vi "HFRR ADV v11.vi"() -> ()   [LabVIEW 2025] (continued)
                  n3634 = property on="TITTLE" class="Str"("Caption.Text"=w4919) -> ()  [unwired: 2 in, 2 out]
                }
                frame 109 {
                  "String 30" <- w4920
                }
                frame 110 {
                  n3635 = property on="Test Date" class="Str"("Caption.Text"=w4921) -> ()  [unwired: 2 in, 2 out]
                  "String 31" <- w4921
                }
                frame 111 {
                  n3636 = property on="Sample ID" class="Str"("Caption.Text"=w4922) -> ()  [unwired: 2 in, 2 out]
                  "String 32" <- w4922
                }
                frame 112 {
                  n3637 = property on="Tested by" class="Str"("Caption.Text"=w4923) -> ()  [unwired: 2 in, 2 out]
                  "String 33" <- w4923
                }
                frame 113 {
                  n3638 = property on="System Configured Printers 2" class="Arr (strict)"("Caption.Text"=w4924) -> ()  [unwired: 2 in, 2 out]
                }
                frame 114 {
                  n3639 = property on="Selected Printer" class="Str"("Caption.Text"=w4925) -> ()  [unwired: 2 in, 2 out]
                }
                frame 115 {
                  n3640 = property on="Select Printer 3" class="DigNum (strict)"("Caption.Text"=w4926) -> ()  [unwired: 2 in, 2 out]
                }
                frame 116 {
                  n3641 = property on="Print" class="Bool (strict)"("Boolean Text.Text"=w4927) -> ()  [unwired: 2 in, 2 out]
                }
                frame 117 {
                  "String 41" <- w4928
                }
                frame 118 {
                  n3642 = property on="tested by" class="Str"("Caption.Text"=w4929) -> ()  [unwired: 2 in, 2 out]
                }
                frame 119 {
                }
                frame 120 {
                  n3643 = property on="Export" class="Bool (strict)"("Boolean Text.Text"=w4930) -> ()  [unwired: 2 in, 2 out]
                }
                frame 121 {
                  n3644 = property on="TEMP INTERCEPT:" class="DigNum (strict)"("Caption.Text"=w4931) -> ()  [unwired: 2 in, 2 out]
                }
                frame 122 {
                  n3645 = property on="AIR TEMP INTERCEPT:" class="DigNum (strict)"("Caption.Text"=w4932) -> ()  [unwired: 2 in, 2 out]
                }
                frame 123 {
                  n3646 = property on="Select File Type" class="Enum (strict)"("Caption.Text"=w4933) -> ()  [unwired: 2 in, 2 out]
                }
                frame 124 {
                  n3647 = property on="s.NO" class="Str"("Caption.Text"=w4934) -> ()  [unwired: 2 in, 2 out]
                  "String 45" <- w4934
                }
                frame 125 {
                  n3648 = property on="trip1 8" class="Bool (strict)"("Boolean Text.Text"=w4935) -> ()  [unwired: 2 in, 2 out]
                }
                frame 126, Default {
                }
              }
            }
          }
          frame #1 {
            w4943 = TRUE ("Visible")
            n3649 = local read "S 91"() -> (w4960:string)
            n3650 = local read "S 90"() -> (w4959:string)
            n3651 = local read "S 88"() -> (w4958:string)
            n3652 = property on="Threshold" class="DigNum (strict)"("Caption.Text"=w4960) -> ()  [unwired: 2 in, 2 out]
            n3653 = property on="File Path" class="Path"("Caption.Text"=w4959) -> ()  [unwired: 2 in, 2 out]
            n3654 = property on="SrvM CP" class="Bool (strict)"("Boolean Text.Text"=w4958) -> ()  [unwired: 2 in, 2 out]
            n3655 = local read "S 71"() -> (w4953:string)
            n3656 = local read "S 86"() -> (w4955:string)
            n3657 = local read "S 85"() -> (w4956:string)
            n3658 = local read "S 87"() -> (w4954:string)
            n3659 = local read "S 84"() -> (w4957:string)
            n3660 = local read "S 103"() -> (w4942:string)
            n3661 = local read "S 104"() -> (w4941:string)
            n3662 = property on="ENTER THE NEW PASSWORD" class="Str"("Caption.Text"=w4954) -> ()  [unwired: 2 in, 2 out]
            n3663 = property on="Password" class="Str"("Caption.Text"=w4956) -> ()  [unwired: 2 in, 2 out]
            n3664 = property on="ENTER CURRENT PASSWORD" class="Str"("Caption.Text"=w4955) -> ()  [unwired: 2 in, 2 out]
            n3665 = property on="EDIT" class="Bool (strict)"("Boolean Text.Text"=w4953) -> ()  [unwired: 2 in, 2 out]
            n3666 = property on="SAVE" class="Bool (strict)"("Boolean Text.Text"=w4957) -> ()  [unwired: 2 in, 2 out]
            n3667 = Build Array(w4942, w4941) -> (w4940:string[])
            n3668 = property on="Heater Button" class="Bool (strict)"("Strings [4]"=w4940) -> ()  [unwired: 2 in, 2 out]
            n3669 = property on="CH-HUMIDITY WET" class="DigNum (strict)"("Caption.Size to Text?"=w4943) -> ()  [unwired: 2 in, 2 out]
            n3670 = property on="CH-HUMIDITY DRY" class="DigNum (strict)"("Caption.Size to Text?"=w4943) -> ()  [unwired: 2 in, 2 out]
            n3671 = property on="CH-POWER -" class="DigNum (strict)"("Caption.Size to Text?"=w4943) -> ()  [unwired: 2 in, 2 out]
            n3672 = property on="CH-HEATER" class="DigNum (strict)"("Caption.Size to Text?"=w4943) -> ()  [unwired: 2 in, 2 out]
            n3673 = property on="CH-POWER +" class="DigNum (strict)"("Caption.Size to Text?"=w4943) -> ()  [unwired: 2 in, 2 out]
            n3674 = local read "S 92"() -> (w4952:string)
            n3675 = local read "S 93"() -> (w4951:string)
            n3676 = local read "S 105"() -> (w4938:string)
            n3677 = local read "S 106"() -> (w4937:string)
            n3678 = Build Array(w4952, w4951) -> ()  [unwired: 1 out]
            n3679 = Build Array(w4938, w4937) -> (w4939:string[])
            n3680 = local read "S 95"() -> (w4949:string)
            n3681 = local read "S 94"() -> (w4950:string)
            n3682 = local read "bs"() -> (w4965:string)
            n3683 = local read "as"() -> (w4966:string)
            n3684 = property on="Humidity" class="Bool (strict)"("Strings [4]"=w4939) -> ()  [unwired: 2 in, 2 out]
            n3685 = Concatenate Strings(w4965, "\r", w4966) -> ()  [unwired: 1 out]
            n3686 = property on="STROKE GAIN :" class="DigNum (strict)"("Caption.Text"=w4949) -> ()  [unwired: 2 in, 2 out]
            n3687 = property on="DISPLACEMENT :" class="DigNum (strict)"("Caption.Text"=w4950) -> ()  [unwired: 2 in, 2 out]
            n3688 = property on="Rh After" class="DigNum (strict)"("Caption.Size to Text?"=TRUE ("Caption.Size to Text")) -> ()  [unwired: 2 in, 2 out]
            n3689 = local read "S 48"() -> (w4989:string)
            n3690 = local read "S 50"() -> (w4987:string)
            n3691 = local read "S 51"() -> (w4986:string)
            n3692 = local read "S 49"() -> (w4988:string)
            n3693 = local read "S 52"() -> (w4985:string)
            n3694 = local read "as"() -> (w4970:string)
            n3695 = local read "bs"() -> (w4971:string)
            n3696 = local read "S 56"() -> (w4984:string)
            n3697 = local read "S 57"() -> (w4983:string)
            n3698 = local read "S 58"() -> (w4982:string)
            n3699 = local read "S 59"() -> (w4981:string)
            n3700 = property on="OPEN" class="Bool (strict)"("Boolean Text.Text"=w4985) -> ()  [unwired: 2 in, 2 out]
            n3701 = property on="OPEN 1" class="Bool (strict)"("Boolean Text.Text"=w4989) -> ()  [unwired: 2 in, 2 out]
            n3702 = property on="OPEN 2" class="Bool (strict)"("Boolean Text.Text"=w4988) -> ()  [unwired: 2 in, 2 out]
            n3703 = property on="OPEN 3" class="Bool (strict)"("Boolean Text.Text"=w4987) -> ()  [unwired: 2 in, 2 out]
            n3704 = property on="OPEN 4" class="Bool (strict)"("Boolean Text.Text"=w4986) -> ()  [unwired: 2 in, 2 out]
            n3705 = Concatenate Strings(w4971, "\r", w4970) -> ()  [unwired: 1 out]
            n3706 = local read "S 102"() -> (w4944:string)
            n3707 = property on="КОФ1" class="DigNum (strict)"("Caption.Text"=w4984) -> ()  [unwired: 2 in, 2 out]
            n3708 = local read "S 98"() -> (w4948:string)
            n3709 = local read "S 99"() -> (w4947:string)
            n3710 = local read "S 100"() -> (w4946:string)
            n3711 = local read "S 101"() -> (w4945:string)
            n3712 = property on="КОФ2" class="DigNum (strict)"("Caption.Text"=w4983) -> ()  [unwired: 2 in, 2 out]
            n3713 = property on="КОФ3" class="DigNum (strict)"("Caption.Text"=w4982) -> ()  [unwired: 2 in, 2 out]
            n3714 = property on="КОФ4" class="DigNum (strict)"("Caption.Text"=w4981) -> ()  [unwired: 2 in, 2 out]
            n3715 = local read "bs"() -> (w4969:string)
            n3716 = local read "as"() -> (w4968:string)
            n3717 = property on="CH-POWER +" class="DigNum (strict)"("Caption.Text"=w4948) -> ()  [unwired: 2 in, 2 out]
            n3718 = property on="CH-POWER -" class="DigNum (strict)"("Caption.Text"=w4947) -> ()  [unwired: 2 in, 2 out]
            n3719 = property on="CH-HEATER" class="DigNum (strict)"("Caption.Text"=w4946) -> ()  [unwired: 2 in, 2 out]
            n3720 = property on="CH-HUMIDITY DRY" class="DigNum (strict)"("Caption.Text"=w4945) -> ()  [unwired: 2 in, 2 out]
            n3721 = property on="CH-HUMIDITY WET" class="DigNum (strict)"("Caption.Text"=w4944) -> ()  [unwired: 2 in, 2 out]
            n3722 = local read "S 60"() -> (w4980:string)
            n3723 = local read "S 54"() -> (w4990:string)
            n3724 = Concatenate Strings(w4969, "\r", w4968) -> ()  [unwired: 1 out]
            n3725 = Concatenate Strings(w4990, w4980) -> ()  [unwired: 1 out]
            n3726 = local read "S 77"() -> (→"String 43":string)
            n3727 = local read "S 76"() -> (w4963:string)
            n3728 = local read "S 78"() -> (w4962:string)
            n3729 = local read "S 71"() -> (w4974:string)
            n3730 = local read "S 66"() -> (w4979:string)
            n3731 = local read "S 67"() -> (w4978:string)
            n3732 = local read "S 68"() -> (w4977:string)
            n3733 = local read "S 69"() -> (w4976:string)
            n3734 = local read "S 70"() -> (w4975:string)
            n3735 = property on="AIR TEMP" class="DigNum (strict)"("Caption.Text"=w4962) -> ()  [unwired: 2 in, 2 out]
            n3736 = property on="Set Strk" class="DigNum (strict)"("Caption.Text"=w4963) -> ()  [unwired: 2 in, 2 out]
            n3737 = property on="FRIC. FORCE :" class="DigNum (strict)"("Caption.Text"=w4979) -> ()  [unwired: 2 in, 2 out]
            n3738 = property on="TEMPERATURE :" class="DigNum (strict)"("Caption.Text"=w4978) -> ()  [unwired: 2 in, 2 out]
            n3739 = property on="SPEED OUT:" class="DigNum (strict)"("Caption.Text"=w4977) -> ()  [unwired: 2 in, 2 out]
            n3740 = property on="AIR TEMPERATURE :" class="DigNum (strict)"("Caption.Text"=w4976) -> ()  [unwired: 2 in, 2 out]
            n3741 = property on="HUMIDITY:" class="DigNum (strict)"("Caption.Text"=w4975) -> ()  [unwired: 2 in, 2 out]
            n3742 = property on="EDIT" class="Bool (strict)"("Boolean Text.Text"=w4974) -> ()  [unwired: 2 in, 2 out]
            n3743 = local read "S 79"() -> (w4961:string)
            n3744 = property on="Stroke" class="DigNum (strict)"("Caption.Text"=w4961) -> ()  [unwired: 2 in, 2 out]
          }
          frame #2 {
          }
        }
        n3745 = local write "Lan flag"(10.0 ("Lan flag")) -> ()
      }
      frame Enabled {
      }
    }
    n3746 = Wait (ms)(milliseconds to wait=u32 2000) -> ()  [unwired: 1 out]
    n3747 = local read "Quit"() -> (w4763:bool)
  }
  n3748 = disable-structure shown="Disabled" {
    frame Disabled {
      n3749 = while {
        tunnel: [w4992] -> _
        i -> [w4992]
        stop <- w4991 continue-if-true
        n3750 = Wait (ms)(milliseconds to wait=u32 50) -> ()  [unwired: 1 out]
        n3751 = stacked-sequence {
          frame #0 {
            # "Controls Text color"
            # "Controls BG color"
            n3752 = property on="FILE" class="Str"("Text.Text Colors:Text Color"="SC  Text") -> ()  [unwired: 2 in, 2 out]
            n3753 = property on="Fuel Discription :" class="Str"("Text.Text Colors:Text Color"="SC  Text") -> ()  [unwired: 2 in, 2 out]
            n3754 = property on="tested by" class="Str"("Text.Text Colors:Text Color"="SC  Text") -> ()  [unwired: 2 in, 2 out]
            n3755 = property on="Remarks :" class="Str"("Text.Text Colors:Text Color"="SC  Text") -> ()  [unwired: 2 in, 2 out]
            n3756 = property class="DigNum (strict)"("Numeric Text.Text Colors:BG Color"="NC BG") -> ()  [unwired: 2 in, 2 out]
            n3757 = property class="DigNum (strict)"("Numeric Text.Text Colors:BG Color"="NC BG") -> ()  [unwired: 2 in, 2 out]
            n3758 = property class="DigNum (strict)"("Numeric Text.Text Colors:BG Color"="NC BG") -> ()  [unwired: 2 in, 2 out]
            n3759 = property class="DigNum (strict)"("Numeric Text.Text Colors:BG Color"="NC BG") -> ()  [unwired: 2 in, 2 out]
            n3760 = property class="DigNum (strict)"("Numeric Text.Text Colors:BG Color"="NC BG") -> ()  [unwired: 2 in, 2 out]
            n3761 = property class="DigNum (strict)"("Numeric Text.Text Colors:BG Color"="NC BG") -> ()  [unwired: 2 in, 2 out]
            n3762 = property class="DigNum (strict)"("Numeric Text.Text Colors:BG Color"="NC BG") -> ()  [unwired: 2 in, 2 out]
            n3763 = property class="DigNum (strict)"("Numeric Text.Text Colors:BG Color"="NC BG") -> ()  [unwired: 2 in, 2 out]
            n3764 = property class="DigNum (strict)"("Numeric Text.Text Colors:BG Color"="NC BG") -> ()  [unwired: 2 in, 2 out]
            n3765 = property class="DigNum (strict)"("Numeric Text.Text Colors:BG Color"="NC BG") -> ()  [unwired: 2 in, 2 out]
            n3766 = property class="DigNum (strict)"("Numeric Text.Text Colors:BG Color"="NC BG") -> ()  [unwired: 2 in, 2 out]
            n3767 = property class="DigNum (strict)"("Numeric Text.Text Colors:BG Color"="NC BG") -> ()  [unwired: 2 in, 2 out]
            n3768 = property on="FILE" class="Str"("Text.Text Colors:BG Color"="SC BG 3") -> ()  [unwired: 2 in, 2 out]
            n3769 = property on="Fuel Discription :" class="Str"("Text.Text Colors:BG Color"="SC BG 3") -> ()  [unwired: 2 in, 2 out]
            n3770 = property on="tested by" class="Str"("Text.Text Colors:BG Color"="SC BG 3") -> ()  [unwired: 2 in, 2 out]
            n3771 = property on="Remarks :" class="Str"("Text.Text Colors:BG Color"="SC BG 3") -> ()  [unwired: 2 in, 2 out]
            n3772 = property class="DigNum (strict)"("Numeric Text.Text Colors:Text Color"="NC Text") -> ()  [unwired: 2 in, 2 out]
            n3773 = property class="DigNum (strict)"("Numeric Text.Text Colors:Text Color"="NC Text") -> ()  [unwired: 2 in, 2 out]
            n3774 = property class="DigNum (strict)"("Numeric Text.Text Colors:Text Color"="NC Text") -> ()  [unwired: 2 in, 2 out]
            n3775 = property class="DigNum (strict)"("Numeric Text.Text Colors:Text Color"="NC Text") -> ()  [unwired: 2 in, 2 out]
            n3776 = property class="DigNum (strict)"("Numeric Text.Text Colors:Text Color"="NC Text") -> ()  [unwired: 2 in, 2 out]
            n3777 = property class="DigNum (strict)"("Numeric Text.Text Colors:Text Color"="NC Text") -> ()  [unwired: 2 in, 2 out]
            n3778 = property class="DigNum (strict)"("Numeric Text.Text Colors:Text Color"="NC Text") -> ()  [unwired: 2 in, 2 out]
            n3779 = property class="DigNum (strict)"("Numeric Text.Text Colors:Text Color"="NC Text") -> ()  [unwired: 2 in, 2 out]
            n3780 = property class="DigNum (strict)"("Numeric Text.Text Colors:Text Color"="NC Text") -> ()  [unwired: 2 in, 2 out]
            n3781 = property class="DigNum (strict)"("Numeric Text.Text Colors:Text Color"="NC Text") -> ()  [unwired: 2 in, 2 out]
            n3782 = property class="DigNum (strict)"("Numeric Text.Text Colors:Text Color"="NC Text") -> ()  [unwired: 2 in, 2 out]
            n3783 = property class="DigNum (strict)"("Numeric Text.Text Colors:Text Color"="NC Text") -> ()  [unwired: 2 in, 2 out]
            n3784 = property class="DigNum (strict)"("Numeric Text.Text Colors:Text Color"="NI Text  2") -> ()  [unwired: 2 in, 2 out]
            n3785 = property class="DigNum (strict)"("Numeric Text.Text Colors:Text Color"="NI Text  2") -> ()  [unwired: 2 in, 2 out]
            n3786 = property class="DigNum (strict)"("Numeric Text.Text Colors:Text Color"="NI Text  2") -> ()  [unwired: 2 in, 2 out]
            n3787 = property class="DigNum (strict)"("Numeric Text.Text Colors:Text Color"="NI Text  2") -> ()  [unwired: 2 in, 2 out]
            n3788 = property class="DigNum (strict)"("Numeric Text.Text Colors:Text Color"="NI Text  2") -> ()  [unwired: 2 in, 2 out]
            n3789 = property class="DigNum (strict)"("Numeric Text.Text Colors:Text Color"="NI Text  2") -> ()  [unwired: 2 in, 2 out]
            n3790 = property class="DigNum (strict)"("Numeric Text.Text Colors:Text Color"="NI Text  2") -> ()  [unwired: 2 in, 2 out]
            n3791 = property class="DigNum (strict)"("Numeric Text.Text Colors:Text Color"="NI Text  2") -> ()  [unwired: 2 in, 2 out]
            n3792 = property class="DigNum (strict)"("Numeric Text.Text Colors:Text Color"="NI Text  2") -> ()  [unwired: 2 in, 2 out]
            n3793 = property class="DigNum (strict)"("Numeric Text.Text Colors:Text Color"="NI Text  2") -> ()  [unwired: 2 in, 2 out]
            n3794 = property class="DigNum (strict)"("Numeric Text.Text Colors:Text Color"="NI Text  2") -> ()  [unwired: 2 in, 2 out]
            n3795 = property class="DigNum (strict)"("Numeric Text.Text Colors:Text Color"="NI Text  2") -> ()  [unwired: 2 in, 2 out]
            n3796 = property class="DigNum (strict)"("Numeric Text.Text Colors:Text Color"="NI Text  2") -> ()  [unwired: 2 in, 2 out]
            n3797 = property class="DigNum (strict)"("Numeric Text.Text Colors:Text Color"="NI Text  2") -> ()  [unwired: 2 in, 2 out]
            n3798 = property class="DigNum (strict)"("Numeric Text.Text Colors:Text Color"="NI Text  2") -> ()  [unwired: 2 in, 2 out]
            n3799 = property class="DigNum (strict)"("Numeric Text.Text Colors:Text Color"="NI Text  2") -> ()  [unwired: 2 in, 2 out]
            n3800 = property on="Coefficient Of Friction" class="XYGraph (strict)"("Plot Area:Colors:FG Color"="GFG  2", "Plot Area:Colors:BG Color"="GBG   2") -> ()  [unwired: 2 in, 2 out]
            n3801 = property on="Humidity ( %RH )" class="XYGraph (strict)"("Plot Area:Colors:FG Color"="GFG  2", "Plot Area:Colors:BG Color"="GBG   2") -> ()  [unwired: 2 in, 2 out]
            n3802 = property on="Air Temperature  ( °C )" class="XYGraph (strict)"("Plot Area:Colors:FG Color"="GFG  2", "Plot Area:Colors:BG Color"="GBG   2") -> ()  [unwired: 2 in, 2 out]
            n3803 = property on="Sample Temperature ( °C )" class="XYGraph (strict)"("Plot Area:Colors:FG Color"="GFG  2", "Plot Area:Colors:BG Color"="GBG   2") -> ()  [unwired: 2 in, 2 out]
            n3804 = property class="DigNum (strict)"("Numeric Text.Text Colors:BG Color"="NI BG 2") -> ()  [unwired: 2 in, 2 out]
            n3805 = property class="DigNum (strict)"("Numeric Text.Text Colors:BG Color"="NI BG 2") -> ()  [unwired: 2 in, 2 out]
            n3806 = property class="DigNum (strict)"("Numeric Text.Text Colors:BG Color"="NI BG 2") -> ()  [unwired: 2 in, 2 out]
            n3807 = property class="DigNum (strict)"("Numeric Text.Text Colors:BG Color"="NI BG 2") -> ()  [unwired: 2 in, 2 out]
            n3808 = property class="DigNum (strict)"("Numeric Text.Text Colors:BG Color"="NI BG 2") -> ()  [unwired: 2 in, 2 out]
            n3809 = property class="DigNum (strict)"("Numeric Text.Text Colors:BG Color"="NI BG 2") -> ()  [unwired: 2 in, 2 out]
            n3810 = property class="DigNum (strict)"("Numeric Text.Text Colors:BG Color"="NI BG 2") -> ()  [unwired: 2 in, 2 out]
            n3811 = property class="DigNum (strict)"("Numeric Text.Text Colors:BG Color"="NI BG 2") -> ()  [unwired: 2 in, 2 out]
            n3812 = property class="DigNum (strict)"("Numeric Text.Text Colors:BG Color"="NI BG 2") -> ()  [unwired: 2 in, 2 out]
            n3813 = property class="DigNum (strict)"("Numeric Text.Text Colors:BG Color"="NI BG 2") -> ()  [unwired: 2 in, 2 out]
            n3814 = property class="DigNum (strict)"("Numeric Text.Text Colors:BG Color"="NI BG 2") -> ()  [unwired: 2 in, 2 out]
            n3815 = property class="DigNum (strict)"("Numeric Text.Text Colors:BG Color"="NI BG 2") -> ()  [unwired: 2 in, 2 out]
            n3816 = property class="DigNum (strict)"("Numeric Text.Text Colors:BG Color"="NI BG 2") -> ()  [unwired: 2 in, 2 out]
            n3817 = property class="DigNum (strict)"("Numeric Text.Text Colors:BG Color"="NI BG 2") -> ()  [unwired: 2 in, 2 out]
            n3818 = property class="DigNum (strict)"("Numeric Text.Text Colors:BG Color"="NI BG 2") -> ()  [unwired: 2 in, 2 out]
            n3819 = property class="DigNum (strict)"("Numeric Text.Text Colors:BG Color"="NI BG 2") -> ()  [unwired: 2 in, 2 out]
            n3820 = property class="Bool"("Colors [4]"="Boolean BC T & BG") -> ()  [unwired: 2 in, 2 out]
            n3821 = property on="Save & Continue" class="Bool (strict)"("Colors [4]"="Boolean BC T & BG") -> ()  [unwired: 2 in, 2 out]
            n3822 = property on="Heater Button" class="Bool (strict)"("Colors [4]"="Boolean BC T & BG") -> ()  [unwired: 2 in, 2 out]
            n3823 = property class="Bool"("Colors [4]"="Boolean BC T & BG") -> ()  [unwired: 2 in, 2 out]
            n3824 = property on="Humidity" class="Bool (strict)"("Colors [4]"="Boolean BC T & BG") -> ()  [unwired: 2 in, 2 out]
            n3825 = property class="Bool (strict)"("Colors [4]"="Boolean BC T & BG") -> ()  [unwired: 2 in, 2 out]
            n3826 = property on="RUN" class="Bool (strict)"("Colors [4]"="Boolean BC T & BG") -> ()  [unwired: 2 in, 2 out]
            n3827 = property on="trip1 8" class="Bool (strict)"("Colors [4]"="Boolean BC T & BG") -> ()  [unwired: 2 in, 2 out]
            n3828 = property class="Bool"("Colors [4]"="Boolean BC T & BG") -> ()  [unwired: 2 in, 2 out]
            n3829 = property class="Bool (strict)"("Colors [4]"="Boolean BC T & BG") -> ()  [unwired: 2 in, 2 out]
            n3830 = property on="OPEN 1" class="Bool (strict)"("Colors [4]"="Boolean BC T & BG 2") -> ()  [unwired: 2 in, 2 out]
            n3831 = property on="OPEN 2" class="Bool (strict)"("Colors [4]"="Boolean BC T & BG 2") -> ()  [unwired: 2 in, 2 out]
            n3832 = property on="OPEN 3" class="Bool (strict)"("Colors [4]"="Boolean BC T & BG 2") -> ()  [unwired: 2 in, 2 out]
            n3833 = property on="OPEN 4" class="Bool (strict)"("Colors [4]"="Boolean BC T & BG 2") -> ()  [unwired: 2 in, 2 out]
            n3834 = property on="OPEN" class="Bool (strict)"("Colors [4]"="Boolean BC T & BG 2") -> ()  [unwired: 2 in, 2 out]
            n3835 = property on="rstv2" class="Bool"("Colors [4]"="Boolean BC T & BG 2") -> ()  [unwired: 2 in, 2 out]
            n3836 = property on="RST CP" class="Bool"("Colors [4]"="Boolean BC T & BG 2") -> ()  [unwired: 2 in, 2 out]
            n3837 = property on="RSTV1 3" class="Bool"("Colors [4]"="Boolean BC T & BG 2") -> ()  [unwired: 2 in, 2 out]
            n3838 = property on="RSTV1 2" class="Bool"("Colors [4]"="Boolean BC T & BG 2") -> ()  [unwired: 2 in, 2 out]
          }
          frame #1 {
          }
        }
        n3839 = local read "Quit"() -> (w4991:bool)
      }
    }
    frame Enabled {
    }
  }
  n3840 = while {
    shift-right: [w5009] -> _
    shift-left: _ -> [w5010]
    shift-right: [w5007] -> _
    shift-left: T17 {"Read Heave and Surge"="", "Bytes at Heave Port"=0.0, "Heave and Surge COM Port:"="COM9", "Com Port 2"="COM7", "Residual Due"="", "Heave COM Status 2"=TRUE, "Heave COM Status"=TRUE, "Port 2"=TRUE, "Sway PPR"=6400.0, "Surge PPR"=6400.0, "Heave PPR"=6400.0, "Sway Pitch"=2.0, "Surge Pitch"=3.0, "Heave Pitch"=4.0, "Sway Pulses/mm"=320.0, "Surge Pulses/mm"=1600.0, "Heave Pulses/mm"=1600.0, "inner loop"=0.0, "Read Heave and Surge 2"="", "String 36"="", "Write S"=FALSE, "WriteCC1"=[""], "Heave COM Loop"=0, "LastCom"="", "EXIT"=FALSE, "Error Heave"={"status"=TRUE, "code"=-1073807343, "source"=""}} -> [w5006]
    shift-right: [w5004] -> _
    shift-left: enum16{"init", "MAIN", "Panel Close"}."init" -> [w5005]
    stop <- w5008 stop-if-true
    n3841 = case shown="\"init\"" w5005 {
      tunnel: w5010 -> [w5024 w5039 w5109 w5111]
      tunnel: [w5018 w5057 w5109 w5111] -> w5009
      tunnel: [_ _ TRUE _] -> w5008
      tunnel: [w5014 w5054 w5107 w5110] -> w5007
      tunnel: w5006 -> [w5021 w5038 w5107 w5110]
      tunnel: [enum16{"init", "MAIN", "Panel Close"}."MAIN" w5032 _ _] -> w5004
      frame "init" {
        n3842 = Bundle By Name(cluster=w5021, "Heave and Surge COM Port:"="C3 :") -> (w5020:T17)
        n3843 = call "Instrument fgv.vi"("Enum"=T27."INIT", "error in (no error) 2"=w5024, "INPUT"=w5020) -> ("error"=w5022:errorcluster, "output"=w5017:T17)  [unwired: 6 in, 1 out]
        n3844 = case shown="No Error" w5022 {
          selector: w5022 -> [w5026 _]
          tunnel: [w5026 w5030] -> w5018
          tunnel: w5017 -> [w5025 w5028]
          tunnel: [w5025 w5027] -> w5015
          frame No Error {
          }
          frame Error {
            n3845 = call "Instrument fgv.vi"("Enum"=T27."ERROR INIT", "INPUT"=w5028) -> ("error"=w5031:errorcluster, "output"=w5027:T17)  [unwired: 7 in, 1 out]
            n3846 = call <vilib>:"Clear Errors.vi"("error in (no error)"=w5031) -> ("error out"=w5030:errorcluster)  [unwired: 5 in, 1 out]
          }
        }
        n3847 = local read "LastCom"() -> (w5013:string)
        n3848 = Unbundle By Name(w5015) -> ("Heave COM Status 2"=→"COM Status" →"Instrument Status":bool, "Error Heave"=→"Error":errorcluster)  [unwired: 1 out]
        n3849 = Bundle By Name(cluster=w5015, "LastCom"=w5013) -> (w5014:T17)
      }
      frame "MAIN" {
        n3850 = Unbundle By Name(w5038) -> ("Com Port 2"=w5059:refnum<visa-resource-name>)
        n3851 = local write "Com Port 4"(w5059) -> ()
        n3852 = local read "C3 :"() -> (w5036:refnum<visa-resource-name>)
        n3853 = Divide(x="Heave PPR", y="Heave Pitch") -> (x/y=→"Heave Pulses/mm":dbl)
        n3854 = Bundle By Name(cluster=w5038, "Heave and Surge COM Port:"=w5036) -> (w5037:T17)
        n3855 = Equal?(x=w5059, y=w5036) -> (x = y?=w5058:bool)
        n3856 = Divide(x="Sway PPR", y="Sway Pitch") -> (x/y=→"Sway Pulses/mm":dbl)
        n3857 = case shown="False" w5058 {
          tunnel: [w5063 w5080] -> w5057
          tunnel: w5039 -> [w5064 w5086]
          tunnel: w5037 -> [w5062 w5084]
          tunnel: [w5061 w5079] -> w5054
          frame False {
            n3858 = call <vilib>:"Clear Errors.vi"("error in (no error)"=w5064) -> ("error out"=w5060:errorcluster)  [unwired: 5 in, 1 out]
            n3859 = call "Instrument fgv.vi"("Enum"=T27."ERROR INIT", "error in (no error) 2"=w5060, "INPUT"=w5062) -> ("error"=w5066:errorcluster, "output"=w5061:T17)  [unwired: 6 in, 1 out]
            n3860 = call <vilib>:"Clear Errors.vi"("error in (no error)"=w5066) -> ("error out"=w5063:errorcluster)  [unwired: 5 in, 1 out]
          }
          frame True {
            n3861 = call "Instrument fgv.vi"("Enum"=T27."READ", "error in (no error) 2"=w5086, "INPUT"=w5084) -> ("error"=w5085:errorcluster, "output"=w5076:T17)  [unwired: 6 in, 1 out]
            n3862 = Bundle By Name(cluster=w5076, "String 36"="String 11") -> (w5075:T17)
            n3863 = case shown="True" "Write S" {
              selector: "Write S" -> [_ w5106]
              tunnel: w5085 -> [w5099 w5105]
              tunnel: [w5099 w5104] -> w5072
              tunnel: w5075 -> [w5098 w5101]
              tunnel: [w5098 w5100] -> w5071
              frame False {
              }
              frame True {
                n3864 = Not(x=w5106) -> (.not. x?=w5102:bool)
                n3865 = local write "Write S"(w5102) -> ()
                n3866 = call "Instrument fgv.vi"("Enum"=T27."MANUAL WRITE", "error in (no error) 2"=w5105, "INPUT"=w5101) -> ("error"=w5104:errorcluster, "output"=w5100:T17)  [unwired: 6 in, 1 out]
              }
            }
            n3867 = Array Size(array="WriteHumidity") -> (size(s)=w5069:i32)
            n3868 = Greater Than 0?(x=w5069) -> (x > 0?=w5067:bool)
            n3869 = call "Instrument fgv.vi"("Enum"=T27."WRITE", "error in (no error) 2"=w5072, "WriteCC1"="WriteHumidity", "INPUT"=w5071) -> ("error"=w5082:errorcluster, "WriteCC1 2"=w5070:string[], "output"=w5081:T17)  [unwired: 5 in]
            n3870 = case shown="True" w5067 {
              tunnel: w5070 -> [_ w5088]
              frame False {
              }
              frame True {
                n3871 = local write "WriteHumidity"(w5088) -> ()
              }
            }
            n3872 = case shown="Error" w5082 {
              selector: w5082 -> [w5089 w5092]
              tunnel: w5081 -> [w5090 w5097]
              tunnel: [w5090 w5096] -> w5079
              tunnel: [w5089 w5094] -> w5080
              frame No Error {
              }
              frame Error {
                n3873 = call <vilib>:"Clear Errors.vi"("error in (no error)"=w5092) -> ("error out"=w5091:errorcluster)  [unwired: 5 in, 1 out]
                n3874 = call "Instrument fgv.vi"("Enum"=T27."ERROR INIT", "error in (no error) 2"=w5091, "INPUT"=w5097) -> ("error"=w5095:errorcluster, "output"=w5096:T17)  [unwired: 6 in, 1 out]
                n3875 = call <vilib>:"Clear Errors.vi"("error in (no error)"=w5095) -> ("error out"=w5094:errorcluster)  [unwired: 5 in, 1 out]
              }
            }
            n3876 = Unbundle By Name(w5079) -> ("LastCom"=→"LastCom":string, "Read Heave and Surge"=→"Read Humidity":string)
          }
        }
        n3877 = Divide(x="Surge PPR", y="Surge Pitch") -> (x/y=→"Surge Pulses/mm":dbl)
        n3878 = Unbundle By Name(w5054) -> ("Heave COM Status 2"=w5056:bool, "Heave COM Status"=w5055:bool, "Error Heave"=w5052:errorcluster, "Bytes at Heave Port"=→"Bytes at Humidity Port":dbl)
        n3879 = Unbundle By Name(w5052) -> ("status"=→"Humidity Port":bool)
        n3880 = Not(x=w5055) -> (.not. x?=w5040:bool)
        n3881 = local write "Error"(w5052) -> ()
        n3882 = Not(x=w5056) -> (.not. x?=w5041:bool)
        n3883 = local write "Instrument Status"(w5040) -> ()
        n3884 = local write "COM Status"(w5041) -> ()
        n3885 = local read "Quit"() -> (w5033:bool)
        n3886 = Select(t=enum16{"init", "MAIN", "Panel Close"}."Panel Close", s=w5033, f=enum16{"init", "MAIN", "Panel Close"}."MAIN") -> (s? t:f=w5032:enum16{"init", "MAIN", "Panel Close"})
      }
      frame "Panel Close" {
      }
      frame Default {
      }
    }
  }
  n3887 = while {
    stop <- w5137 stop-if-true
    n3888 = local read "Read Humidity"() -> (w5118:string)
    n3889 = call <vilib>:"High Resolution Polling Wait.vi"("seconds to wait"=0.1) -> ()  [unwired: 10 in, 1 out]
    n3890 = Spreadsheet String To Array(delimiter (Tab)=",", format string="", spreadsheet string=w5118, array type (2D Dbl)=string[] []) -> (array=w5132:string[])
    n3891 = for {
      tunnel: w5132 -> [w5142] mode=indexing
      tunnel: string[] ["STATE;", "SET;", "RH;", "T;", "AMB_RH;", "AMB_T;", "PUMP;", "FAN_IN;", "FAN_OUT;", "DEHUM;", "CURRENT;", "STALL;"] -> [w5141] mode=indexing
      tunnel: [w5140] -> w5131 mode=indexing
      n3892 = Match Pattern(string=w5142, regular expression=w5141) -> (after substring=w5140:string)  [unwired: 1 in, 3 out]
    }
    n3893 = Index Array(array=w5131) -> (element #1=→"STATE :":string, element #2=→"SET :":string, element #3=w5120:string, element #4=→"T :":string, element #5=w5117:string, element #6=→"AMB_T :":string, element #7=→"PUMP :":string, element #8=→"FAN_IN :":string, element #9=→"FAN_OUT :":string, element #10=→"DEHUM :":string, element #11=→"CURRENT :":string, element #12=→"STALL :":string)  [unwired: 12 in]
    "RH :" <- w5120
    "AMB_RH :" <- w5117
    n3894 = Fract/Exp String To Number(string=w5120) -> (number=w5112:dbl)  [unwired: 3 in, 1 out]
    n3895 = Fract/Exp String To Number(string=w5117) -> (number=w5116:dbl)  [unwired: 3 in, 1 out]
    n3896 = local write "Ambient Humidity :"(w5116) -> ()
    n3897 = Equal?(x=w5112, y=0.0) -> (x = y?=w5114:bool)
    n3898 = case shown="True" w5114 {
      tunnel: [w5138 w5139] -> w5113
      tunnel: w5112 -> [w5138 _]
      frame False {
        (unwired) 0.0
        "Humidity temp" <- w5138
      }
      frame True {
        n3899 = local read "Humidity temp"() -> (w5139:dbl)
      }
    }
    "RH Numeric:" <- w5113
    n3900 = local read "Quit"() -> (w5137:bool)
  }
  n3901 = disable-structure shown="Disabled" {
    frame Disabled {
      n3902 = while {
        tunnel: [w5376] -> _
        i -> [w5376]
        stop <- w5373 stop-if-true
        n3903 = local read "powstat"() -> (w5374:bool)
        n3904 = case shown="True" w5374 {
          frame False {
          }
          frame True {
            n3905 = local read "RUN"() -> (w5377:bool)
            n3906 = case shown="True" w5377 {
              frame False {
                w5407 = 65.0 ("y")
                n3907 = local read "Set Hz"() -> (w5435:dbl)
                n3908 = local read "NORMAL LOAD"() -> (w5436:dbl)
                n3909 = Multiply(x=w5435, y=60.0) -> (x*y=w5442:dbl)
                n3910 = Multiply(x=1.2 ("y"), y=0.949) -> (x*y=w5411:dbl)
                n3911 = Multiply(x=1.2 ("y"), y=0.8166) -> (x*y=w5415:dbl)
                n3912 = Multiply(x=1.2 ("y"), y=0.851) -> (x*y=w5410:dbl)
                n3913 = local read "FF 2"() -> (w5434:dbl)
                n3914 = Absolute Value(x=w5442) -> (abs(x)=w5440:dbl)
                n3915 = local read "Stroke"() -> (w5409:dbl)
                n3916 = Less?(x=w5409, y=w5415) -> (x < y?=w5412:bool)
                n3917 = In Range and Coerce(upper limit=w5411, x=w5409, lower limit=w5410) -> (In Range?=w5413:bool)  [unwired: 1 out]
                n3918 = case shown="13.." w5434 {
                  tunnel: [1 2 3] -> w5432
                  frame 0..10, Default {
                    # "Normal"
                  }
                  frame 11, 12 {
                  }
                  frame 13.. {
                  }
                }
                "FF STATE" <- w5432
                n3919 = local read "TEMP"() -> (w5395:dbl)
                n3920 = case shown="3601.." w5440 {
                  tunnel: [1 2 3] -> w5438
                  frame 0..3000, Default {
                    # "Normal"
                  }
                  frame 3001..3600 {
                  }
                  frame 3601.. {
                  }
                }
                n3921 = case shown="11.." w5436 {
                  tunnel: [1 3] -> w5437
                  frame 1..10, Default {
                  }
                  frame 11.. {
                  }
                }
                "NL STATE" <- w5437
                n3922 = Multiply(x=1.2 ("y"), y=0.95) -> (x*y=w5425:dbl)
                n3923 = Multiply(x=w5407, y=0.954) -> (x*y=w5399:dbl)
                n3924 = Or(x=w5412, y=w5413) -> (x .or. y?=w5414:bool)
                n3925 = Greater Or Equal?(x=w5409, y=w5425) -> (x >= y?=w5422:bool)
                n3926 = Multiply(x=w5407, y=0.99) -> (x*y=w5396:dbl)
                n3927 = Greater Or Equal?(x=w5395, y=w5396) -> (x >= y?=w5401:bool)
                n3928 = Greater Or Equal?(x=w5395, y=w5399) -> (x >= y?=w5398:bool)
                n3929 = case shown="0, 1, Default" w5409 {
                  tunnel: [1 3] -> w5426
                  frame 0, 1, Default {
                  }
                  frame 2.. {
                  }
                }
                n3930 = case shown="True" w5422 {
                  tunnel: [1 3] -> w5427
                  frame False {
                  }
                  frame True {
                  }
                }
                n3931 = case shown="True" w5414 {
                  tunnel: [1 2] -> w5428
                  frame False {
                  }
                  frame True {
                  }
                }
                n3932 = case shown="..0" w5395 {
                  tunnel: [2 3 3 1] -> w5402
                  frame 61, 62 {
                  }
                  frame 63.. {
                  }
                  frame ..0 {
                  }
                  frame 10..60, Default {
                  }
                }
                n3933 = case shown="True" w5401 {
                  tunnel: [1 3] -> w5403
                  frame False {
                  }
                  frame True {
                  }
                }
                n3934 = Number To Decimal String(number=w5438) -> (decimal integer string=w5439:string)  [unwired: 1 in]
                n3935 = case shown="True" w5398 {
                  tunnel: [1 2] -> w5404
                  frame False {
                  }
                  frame True {
                  }
                }
                n3936 = Number To Decimal String(number=1) -> (decimal integer string=→"Air temp":string)  [unwired: 1 in]
                n3937 = Number To Decimal String(number=w5432) -> (decimal integer string=→"ff_st":string)  [unwired: 1 in]
                n3938 = local write "sp_st"(w5439) -> ()
                n3939 = Number To Decimal String(number=w5437) -> (decimal integer string=→"nl_st":string)  [unwired: 1 in]
                n3940 = Build Array(w5402, w5403, w5404) -> (w5405:i32[])
                n3941 = Build Array(w5426, w5427, w5428) -> (w5429:i32[])
                n3942 = Array Max & Min(array=w5405) -> (max value=w5406:i32)  [unwired: 3 out]
                n3943 = Array Max & Min(array=w5429) -> (max value=w5430:i32)  [unwired: 3 out]
                n3944 = Number To Decimal String(number=w5406) -> (decimal integer string=w5394:string)  [unwired: 1 in]
                n3945 = Number To Decimal String(number=w5430) -> (decimal integer string=→"Stroke Ln 2":string)  [unwired: 1 in]
                n3946 = local write "temp_st"(w5394) -> ()
              }
              frame True {
                w5492 = 65.0 ("y")
                # "Healthy -1\nWarning -2\nError -3"
                n3947 = local read "TEMP"() -> (w5503:dbl)
                n3948 = local read "NORMAL LOAD"() -> (w5507:dbl)
                n3949 = local read "Set Hz"() -> (w5505:dbl)
                n3950 = Multiply(x=1.2 ("y"), y=0.949) -> (x*y=w5487:dbl)
                n3951 = Multiply(x=1.2 ("y"), y=0.8166) -> (x*y=w5483:dbl)
                n3952 = Multiply(x=1.2 ("y"), y=0.851) -> (x*y=w5488:dbl)
                n3953 = Multiply(x=w5492, y=0.954) -> (x*y=w5499:dbl)
                n3954 = Multiply(x=w5492, y=0.99) -> (x*y=w5502:dbl)
                n3955 = Greater Or Equal?(x=w5503, y=w5502) -> (x >= y?=w5497:bool)
                n3956 = Multiply(x=w5505, y=60.0) -> (x*y=w5511:dbl)
                n3957 = Greater Or Equal?(x=w5503, y=w5499) -> (x >= y?=w5500:bool)
                n3958 = local read "FF 2"() -> (w5506:dbl)
                n3959 = local read "Stroke"() -> (w5489:dbl)
                n3960 = Less?(x=w5489, y=w5483) -> (x < y?=w5486:bool)
                n3961 = In Range and Coerce(upper limit=w5487, x=w5489, lower limit=w5488) -> (In Range?=w5485:bool)  [unwired: 1 out]
                n3962 = Absolute Value(x=w5511) -> (abs(x)=w5509:dbl)
                n3963 = case shown="63.." w5503 {
                  tunnel: [2 3 3 1] -> w5496
                  frame 61, 62 {
                  }
                  frame 63.. {
                  }
                  frame ..0 {
                  }
                  frame 10..60, Default {
                  }
                }
                n3964 = case shown="True" w5497 {
                  tunnel: [1 3] -> w5495
                  frame False {
                  }
                  frame True {
                  }
                }
                n3965 = case shown="True" w5500 {
                  tunnel: [1 2] -> w5494
                  frame False {
                  }
                  frame True {
                  }
                }
                n3966 = Multiply(x=1.2 ("y"), y=0.95) -> (x*y=w5473:dbl)
                n3967 = case shown="1..10, Default" w5507 {
                  tunnel: [1 3] -> w5514
                  frame 1..10, Default {
                  }
                  frame 11.. {
                  }
                }
                n3968 = case shown="0..10, Default" w5506 {
                  tunnel: [1 2 3] -> w5513
                  frame 0..10, Default {
                  }
                  frame 11, 12 {
                  }
                  frame 13.. {
                  }
                }
                n3969 = case shown="3601.." w5509 {
                  tunnel: [1 2 3] -> w5508
                  frame 0..3000, Default {
                    # "Normal"
                  }
                  frame 3001..3600 {
                  }
                  frame 3601.. {
                  }
                }
                n3970 = Or(x=w5486, y=w5485) -> (x .or. y?=w5484:bool)
                n3971 = Greater Or Equal?(x=w5489, y=w5473) -> (x >= y?=w5476:bool)
                n3972 = case shown="0, 1, Default" w5489 {
                  tunnel: [1 3] -> w5472
                  frame 0, 1, Default {
                  }
                  frame 2.. {
                  }
                }
                n3973 = case shown="True" w5476 {
                  tunnel: [1 3] -> w5471
                  frame False {
                  }
                  frame True {
                  }
                }
                n3974 = case shown="True" w5484 {
                  tunnel: [1 2] -> w5470
                  frame False {
                  }
                  frame True {
                  }
                }
                n3975 = Build Array(w5496, w5495, w5494) -> (w5493:i32[])
                n3976 = Number To Decimal String(number=w5508) -> (decimal integer string=→"sp_st":string)  [unwired: 1 in]
                n3977 = Array Max & Min(array=w5493) -> (max value=w5490:i32)  [unwired: 3 out]
                "TEMP STATE" <- w5490
                n3978 = Number To Decimal String(number=w5514) -> (decimal integer string=w5517:string)  [unwired: 1 in]
                n3979 = Number To Decimal String(number=w5513) -> (decimal integer string=w5515:string)  [unwired: 1 in]
                n3980 = Number To Decimal String(number=w5490) -> (decimal integer string=→"temp_st":string)  [unwired: 1 in]
                n3981 = Build Array(w5472, w5471, w5470) -> (w5469:i32[])
                n3982 = local write "nl_st"(w5517) -> ()
                n3983 = local write "ff_st"(w5515) -> ()
                n3984 = Number To Decimal String(number=1) -> (decimal integer string=w5512:string)  [unwired: 1 in]
                n3985 = Array Max & Min(array=w5469) -> (max value=w5468:i32)  [unwired: 3 out]
                n3986 = local write "Air temp"(w5512) -> ()
                n3987 = Number To Decimal String(number=w5468) -> (decimal integer string=w5467:string)  [unwired: 1 in]
                n3988 = local write "Stroke Ln 2"(w5467) -> ()
              }
            }
            n3989 = local read "Stroke Ln 2"() -> (w5379:string)
            n3990 = local read "nl_st"() -> (w5385:string)
            n3991 = local read "ff_st"() -> (w5382:string)
            n3992 = local read "sp_st"() -> (w5383:string)
            n3993 = local read "temp_st"() -> (w5384:string)
            n3994 = local read "Air temp"() -> (w5378:string)
            n3995 = Replace Array Subset(array="in", new element #1=w5385, index #1=1 ("index"), new element #2=w5382, index #2=2 ("index"), new element #3=w5384, index #3=3 ("index"), new element #4=w5383, index #4=4 ("index"), new element #5=w5379, index #5=5 ("index"), new element #6=w5378, index #6=6 ("index"), new element #7="Sensor State" ("new element/subarray"), index #7=0 ("index")) -> (→"out":string[])
          }
        }
        n3996 = Wait (ms)(milliseconds to wait=u32 10) -> ()  [unwired: 1 out]
        n3997 = local read "Quit"() -> (w5373:bool)
      }
      n3998 = while {
        stop <- w5348 stop-if-true
        n3999 = local read "run replace"() -> (w5350:bool)
        n4000 = Wait (ms)(milliseconds to wait=u32 100) -> ()  [unwired: 1 out]
        n4001 = Equal?(x="FLAG 2", y=0.0) -> (x = y?=w5351:bool)
        n4002 = case shown="True" w5351 {
          frame False {
          }
          frame True {
            n4003 = local write "FLAG 2"(100.0 ("FLAG 2")) -> ()
            n4004 = call <vilib>:"Read Characters From File.vi"("file path (dialog if empty)"=path "C:/LAB-IQ-NXT/WO 2449 TT.sig", "convert eol? (no:F)"=FALSE ("append to file? (new file:F)")) -> ("character string"=w5354:string)  [unwired: 4 in, 3 out]
            n4005 = call <vilib>:"Read Characters From File.vi"("file path (dialog if empty)"=path "C:/LAB-IQ-NXT/WO 2449 TRH.sig", "convert eol? (no:F)"=FALSE ("append to file? (new file:F)")) -> ("character string"=w5355:string)  [unwired: 4 in, 3 out]
            n4006 = Decimal String To Number(string=w5354) -> (number=w5356:i32)  [unwired: 2 in, 1 out]
            n4007 = local write "Total No. of Tests"(w5356) -> ()
            n4008 = Decimal String To Number(string=w5355) -> (number=w5359:i32)  [unwired: 2 in, 1 out]
            n4009 = local write "SEN.RUN HRS"(w5359) -> ()
          }
        }
        n4010 = case shown="True" w5350 {
          frame False {
          }
          frame True {
            n4011 = Equal?(x="FLAG 4", y=0.0) -> (x = y?=w5363:bool)
            n4012 = case shown="False" w5363 {
              frame False {
                n4013 = Get Date/Time In Seconds() -> (seconds since 1Jan1904=w5369:timestamp)
                n4014 = local read "START 3"() -> (w5367:dbl)
                n4015 = To Double Precision Float(number=w5369) -> (double precision float=w5368:dbl)
                n4016 = Subtract(x=w5368, y=w5367) -> (x-y=→"SENSOR TIME":dbl)
              }
              frame True {
                n4017 = Get Date/Time In Seconds() -> (seconds since 1Jan1904=w5371:timestamp)
                n4018 = local write "FLAG 4"(100.0 ("FLAG")) -> ()
                n4019 = To Double Precision Float(number=w5371) -> (double precision float=→"START 3":dbl)
              }
            }
          }
        }
        n4020 = local read "Quit"() -> (w5348:bool)
      }
      n4021 = while {
        shift-right: [w5148] -> _
        shift-left: _ -> [w5149]
        tunnel: [w5144] -> _
        i -> [w5144]
        stop <- w5143 stop-if-true
        n4022 = Wait (ms)(milliseconds to wait=u32 50 ("Refresh Rate (ms)")) -> ()  [unwired: 1 out]
        n4023 = local read "Json End Flg"() -> (w5145:bool)
        n4024 = Not(x="Upld AR 2") -> ()  [unwired: 1 out]
        n4025 = local read "Upld AR 2"() -> (w5146:bool)
        n4026 = call "Elapsed Time9"("Time Target (s)"="Sen.Upload Rate (s)", "Reset"=FALSE, "Auto Reset"=TRUE) -> ("Time has Elapsed"=w5155:bool)  [unwired: 9 in, 7 out]
        n4027 = Or(x=w5155, y=w5145) -> (x .or. y?=w5151:bool)
        n4028 = case shown="True" w5151 {
          frame False {
          }
          frame True {
            w5247 = "\"SensorName\":\"" ("string")
            w5217 = " \"},{"
            w5242 = "\",\"SensorState\":\""
            w5244 = "\",\"SensorModelNumber\":\"" ("string")
            w5243 = "\",\"SensorRuntimeHours\":\"" ("string")
            n4029 = local read "model num"() -> (w5241:string[])
            n4030 = local read "Sensor name"() -> (w5260:string[])
            n4031 = local read "run"() -> (w5231:string[])
            n4032 = local read "SENSOR TIME"() -> (w5187:dbl)
            n4033 = local read "out"() -> (w5180:string[])
            n4034 = local read "Total No. of Tests"() -> (w5185:dbl)
            n4035 = Select(t=60.0, s="Run test 3", f=3600.0) -> (s? t:f=w5195:dbl)
            n4036 = Index Array(array=w5241, index #1=1 ("index")) -> (element #1=w5240:string, element #2=w5239:string, element #3=w5238:string, element #4=w5237:string, element #5=w5236:string, element #6=w5235:string)  [unwired: 5 in]
            n4037 = Index Array(array=w5231, index #1=1 ("index")) -> (element #1=w5230:string, element #2=w5229:string, element #3=w5228:string, element #4=w5227:string, element #5=w5226:string, element #6=w5225:string)  [unwired: 5 in]
            n4038 = Index Array(array=w5260, index #1=1 ("index")) -> (element #1=w5259:string, element #2=w5258:string, element #3=w5257:string, element #4=w5256:string, element #5=w5246:string, element #6=w5245:string)  [unwired: 5 in]
            n4039 = Index Array(array=w5180, index #1=1 ("index")) -> (element #1=w5212:string, element #2=w5211:string, element #3=w5210:string, element #4=w5209:string, element #5=w5208:string, element #6=w5207:string)  [unwired: 5 in]
            n4040 = local read "SEN.RUN HRS"() -> (w5183:dbl)
            n4041 = Divide(x=w5187, y=w5195) -> (x/y=w5194:dbl)
            n4042 = Increment(x=w5194) -> (x+1=w5190:dbl)
            n4043 = Number To Decimal String(number=w5190) -> (decimal integer string=→"run hrs":string)  [unwired: 1 in]
            n4044 = Divide(x=w5183, y=3600.0 ("f")) -> (x/y=w5178:dbl)
            n4045 = Round To Nearest(number=w5178) -> (nearest integer value=w5176:dbl)
            n4046 = Number To Decimal String(number=w5176) -> (decimal integer string=w5177:string)  [unwired: 1 in]
            n4047 = Number To Decimal String(number=w5185) -> (decimal integer string=w5186:string)  [unwired: 1 in]
            n4048 = local read "Model No"() -> (w5191:string)
            n4049 = local read "UUID"() -> (w5286:string)
            n4050 = local read "Serial No"() -> (w5290:string)
            n4051 = local read "Secret Key"() -> (w5291:string)
            n4052 = Concatenate Strings("\",\"MachineSerialNumber\":\"" ("string"), w5290) -> (w5294:string)
            n4053 = Concatenate Strings("\",\"ModelNumber\":\"" ("string"), w5191) -> (w5192:string)
            n4054 = Concatenate Strings("\",\"MachineRuntimeHours\":\"" ("string"), w5177) -> (w5295:string)
            n4055 = Concatenate Strings("\",\"MachineRuntimeCycles\":\"", w5186) -> (w5288:string)
            n4056 = Concatenate Strings(w5244, w5240) -> (w5274:string)
            n4057 = Concatenate Strings(w5243, w5230) -> (w5275:string)
            n4058 = Concatenate Strings(w5242, w5212) -> (w5273:string)
            n4059 = Concatenate Strings(w5294, w5192, w5295, w5288) -> (w5297:string)
            n4060 = Concatenate Strings(w5244, w5239) -> (w5271:string)
            n4061 = Concatenate Strings(w5243, w5229) -> (w5270:string)
            n4062 = Concatenate Strings(w5242, w5211) -> (w5272:string)
            n4063 = Concatenate Strings(w5244, w5238) -> (w5266:string)
            n4064 = Concatenate Strings(w5243, w5228) -> (w5267:string)
            n4065 = Concatenate Strings(w5242, w5210) -> (w5265:string)
            n4066 = Concatenate Strings(w5244, w5237) -> (w5263:string)
            n4067 = Concatenate Strings(w5243, w5227) -> (w5262:string)
            n4068 = Concatenate Strings(w5242, w5209) -> (w5264:string)
            n4069 = Concatenate Strings(w5274, w5275, w5273) -> (w5276:string)
            n4070 = Concatenate Strings(w5244, w5236) -> (w5253:string)
            n4071 = Concatenate Strings(w5243, w5226) -> (w5254:string)
            n4072 = Concatenate Strings(w5244, w5235) -> (w5250:string)
            n4073 = Concatenate Strings(w5243, w5225) -> (w5249:string)
            n4074 = Concatenate Strings(w5242, w5208) -> (w5252:string)
            n4075 = Concatenate Strings(w5242, w5207) -> (w5251:string)
            n4076 = Concatenate Strings("{\"SecretKey\":\"", w5291, w5297, "\",\"UUID\" : \"", w5286, "\",\"SensorInformation\":", "[{" ("string")) -> (w5224:string)
            n4077 = Concatenate Strings(w5271, w5270, w5272) -> (w5269:string)
            n4078 = Concatenate Strings(w5266, w5267, w5265) -> (w5268:string)
            n4079 = Concatenate Strings(w5263, w5262, w5264) -> (w5261:string)
            n4080 = Concatenate Strings(w5253, w5254, w5252) -> (w5255:string)
            n4081 = Concatenate Strings(w5250, w5249, w5251) -> (w5248:string)
            n4082 = Concatenate Strings(w5247, w5259, w5276, w5217) -> (w5223:string)
            n4083 = Concatenate Strings(w5247, w5258, w5269, w5217) -> (w5222:string)
            n4084 = Concatenate Strings(w5247, w5257, w5268, w5217) -> (w5221:string)
            n4085 = Concatenate Strings(w5247, w5256, w5261, w5217) -> (w5220:string)
            n4086 = Concatenate Strings(w5247, w5246, w5255, w5217) -> (w5219:string)
            n4087 = Concatenate Strings(w5247, w5245, w5248, "\"}" ("string")) -> (w5218:string)
            n4088 = Concatenate Strings(w5224, w5223, w5222, w5221, w5220, w5219, w5218, "]}" ("string")) -> (w5215:string)
            n4089 = local read "SEN.RUN HRS"() -> (w5182:dbl)
            n4090 = disable-structure shown="Disabled" {
              frame Disabled {
                n4091 = local read "state"() -> (w5301:string[])
                n4092 = Delete From Array(array=w5301, index=0) -> (array with subset deleted=w5299:string[])  [unwired: 1 in, 1 out]
                n4093 = for {
                  N: 6 -> [_]
                  tunnel: w5299 -> [w5312] mode=indexing
                  tunnel: [w5311] -> w5298 mode=indexing
                  n4094 = Equal?(x=w5312, y="Warning") -> (x = y?=w5308:bool)
                  n4095 = Equal?(x=w5312, y="Healthy") -> (x = y?=w5305:bool)
                  n4096 = Select(t="2" ("y"), s=w5308, f="3" ("y")) -> (s? t:f=w5303:string)
                  n4097 = Select(t="1" ("y"), s=w5305, f=w5303) -> (s? t:f=w5311:string)
                }
                "state1" <- w5298
              }
              frame Enabled {
              }
            }
            n4098 = stacked-sequence {
              tunnel: w5215 -> [w5323 _ _]
              tunnel: [_ _ w5339] -> _
              frame #0 {
                (unwired) FALSE ("convert eol (F)")
                w5325 = enum16{"start", "end", "current"}."start" ("pos mode (0:2)")
                n4099 = local read "Path"() -> (w5319:path)
                n4100 = Path To String(path=w5319) -> (string=w5331:string)
                n4101 = Concatenate Strings(w5331, "\\", "Sensor File Name") -> (w5332:string)
                n4102 = local write "standard output 2"(" ") -> ()
                n4103 = String To Path(string=w5332) -> (path=w5322:path)
                n4104 = call <vilib>:"Open_Create_Replace File.vi"("advisory dialog? (display:T)"=FALSE, "function (open:0)"=T28."create or replace", "file path"=w5322) -> ("error out"=w5335:errorcluster, "refnum"=w5334:refnum<file>)  [unwired: 5 in, 2 out]
                n4105 = Set File Position(refnum=w5334, from (0:start)=w5325, error in=w5335) -> (refnum out=w5315:refnum<file>, error out=w5314:errorcluster)  [unwired: 1 in]
                n4106 = Write to Binary File(file (use dialog)=w5315, data=" ", error in=w5314, 5:FALSE ("prepend array or string size? (T)")) -> (refnum out=w5326:refnum<file>, error out=w5327:errorcluster)  [unwired: 2 in, 1 out]
                n4107 = Set File Position(offset (in bytes) (0)=w5325, refnum=w5326, error in=w5327) -> (refnum out=w5318:refnum<file>, error out=w5317:errorcluster)  [unwired: 1 in]
                n4108 = Write to Binary File(file (use dialog)=w5318, data=w5323, error in=w5317, 5:FALSE ("prepend array or string size? (T)")) -> (error out=w5321:errorcluster)  [unwired: 2 in, 2 out]
                n4109 = flat-sequence {
                  tunnel: w5322 -> [w5337]
                  tunnel: w5321 -> [_]
                  frame #0 {
                    n4110 = call <vilib>:"Read Characters From File.vi"("file path (dialog if empty)"=w5337) -> ("character string"=→"Sensor Health JSON string":string)  [unwired: 5 in, 3 out]
                  }
                }
                "SinglePoint  2" <- w5323
              }
              frame #1 {
              }
              frame #2 {
                (unwired) "\"Stored\": true" ("string")
                n4111 = call <vilib>:"System Exec.vi"("run minimized? (F)"=TRUE, "wait until completion? (T)"=TRUE, "working directory"=path "C:/LAB-IQ-NXT", "command line"="C:\\LAB-IQ-NXT\\JPostH.bat") -> ("standard error"=→"Respose From Server 2":string, "standard output"=w5342:string)  [unwired: 4 in, 2 out]
                "standard output 2" <- w5342
                n4112 = Match Pattern(string=w5342, regular expression="JSONH Check String") -> (match substring=w5340:string, offset past match=w5339:i32)  [unwired: 1 in, 2 out]
                n4113 = Equal?(x=w5340, y="JSONH Check String") -> (x = y?=→"Upload \nConfirmed 2":bool)
              }
            }
            n4114 = Divide(x=w5182, y=3600.0 ("f")) -> (x/y=w5175:dbl)
            n4115 = local read "run time"() -> (w5232:string[])
            n4116 = Round To Nearest(number=w5175) -> (nearest integer value=w5174:dbl)
            n4117 = Number To Decimal String(number=w5174) -> (decimal integer string=w5173:string)  [unwired: 1 in]
            n4118 = Index Array(array="Sensor Information", index (col) #1=0 ("disabled index (col)"), index (col) #2=1 ("index (col)"), index (col) #3=2 ("index (col)"), index (col) #4=3 ("index (col)")) -> (element #1=→"Sensor name":string[], element #2=→"model num":string[], element #3=→"run time":string[], element #4=→"state":string[])  [unwired: 4 in]
            n4119 = Insert Into Array(array=w5232, index=1, new element #1=w5173, new element #2=w5173, new element #3=w5173, new element #4=w5173, new element #5=w5173, new element #6=w5173) -> (w5197:string[])
            "run" <- w5197
            n4120 = local read "out"() -> (w5179:string[])
            n4121 = local read "Sensor Information"() -> (w5199:string[][])
            n4122 = Replace Array Subset(array=w5199, new element #1=w5197, index (col) #1=2 ("disabled index (col)"), new element #2=w5179, index (col) #2=3 ("index (col)")) -> (w5198:string[][])  [unwired: 2 in]
            n4123 = local write "Sensor Information"(w5198) -> ()
          }
        }
        n4124 = case shown="True" w5146 {
          frame False {
          }
          frame True {
            n4125 = Equal?(x="FLAG", y=0.0) -> (x = y?=w5163:bool)
            n4126 = case shown="False" w5163 {
              frame False {
                n4127 = Get Date/Time In Seconds() -> (seconds since 1Jan1904=w5169:timestamp)
                n4128 = local read "START 2"() -> (w5167:dbl)
                n4129 = To Double Precision Float(number=w5169) -> (double precision float=w5168:dbl)
                n4130 = Subtract(x=w5168, y=w5167) -> (x-y=→"SENSOR TIME  2":dbl)
              }
              frame True {
                n4131 = Get Date/Time In Seconds() -> (seconds since 1Jan1904=w5171:timestamp)
                n4132 = To Double Precision Float(number=w5171) -> (double precision float=→"START 2":dbl)
                n4133 = local write "FLAG"(100.0 ("FLAG")) -> ()
              }
            }
          }
        }
        n4134 = disable-structure shown="Disabled" {
          disable-tunnel: w5149 -> [w5158 _]
          disable-tunnel: [w5157 _] -> w5148
          frame Disabled {
            n4135 = local read "Json St Flg"() -> (w5156:bool)
            n4136 = case shown="True" w5156 {
              tunnel: w5158 -> [w5159 w5161]
              tunnel: [w5159 w5160] -> w5157
              frame False {
              }
              frame True {
                n4137 = Increment(x=w5161) -> (x+1=w5160:dbl)
                "T cycle" <- w5160
                n4138 = local write "Json St Flg"(FALSE ("Json St Flg")) -> ()
              }
            }
          }
          frame Enabled {
          }
        }
        n4139 = local read "Quit"() -> (w5143:bool)
      }
    }
    frame Enabled {
    }
  }
  n4140 = stacked-sequence {
    tunnel: [w5541] -> w35
    frame #0 {
      w5541 = FALSE ("Upload \nConfirmed")
      n4141 = local write "Upload \nConfirmed"(w5541) -> ()
      n4142 = local write "St Str"("") -> ()
    }
  }
  n4143 = disable-structure shown="Disabled" {
    disable-tunnel: w35 -> [w5542 _]
    frame Disabled {
      n4144 = case shown="True" {
        selector: _ -> [_ _]
        tunnel: w5542 -> [_ w5543]
        frame False {
        }
        frame True {
          n4145 = while {
            tunnel: [w5549] -> _
            tunnel: w5543 -> [_]
            i -> [w5549]
            stop <- w5544 stop-if-true
            n4146 = local read "Json End Flg"() -> (w5548:bool)
            n4147 = Wait (ms)(milliseconds to wait=u32 20 ("Refresh Rate (ms)")) -> ()  [unwired: 1 out]
            n4148 = local read "refresh flag"() -> (w5545:bool)
            n4149 = local read "RUN"() -> (w5546:bool)
            n4150 = And(x=w5546, y=w5545) -> (x .and. y?=w5547:bool)
            n4151 = Or(x=w5547, y=w5548) -> (x .or. y?=w5550:bool)
            "AR Led" <- w5550
            n4152 = case shown="True" w5550 {
              frame False {
              }
              frame True {
                w5567 = "\",\""
                n4153 = local read "UUID"() -> (w5565:string)
                n4154 = local write "refresh flag"(FALSE ("refresh flag")) -> ()
                n4155 = local read "time"() -> (w5554:dbl)
                n4156 = Multiply(x=w5554, y=60.0) -> (x*y=w5553:dbl)
                n4157 = Concatenate Strings("UUID\" : \"", w5565, "\"}") -> (w5568:string)
                n4158 = Number To Fractional String(number=w5553, width (-)=i16 10, precision (6)=i16 4) -> (F-format string=w5582:string)  [unwired: 1 in]
                n4159 = Concatenate Strings("{", "\"Time\":\"", w5582, w5567) -> (w5577:string)
                n4160 = stacked-sequence {
                  tunnel: w5567 -> [w5630 w5638 w5645 w5653 w5661 w5670 w5677]
                  tunnel: [w5631 _ _ _ _ _ _] -> w5581
                  tunnel: [_ w5639 _ _ _ _ _] -> w5580
                  tunnel: [_ _ w5646 _ _ _ _] -> w5579
